vi "1_OnDemand.vi"() -> ()   [LabVIEW 2020]
uses:
  <vilib>/Instr/_visa.llb/VISA Configure Serial Port (Instr).vi
  <vilib>/Analysis/NI_AALBase.lvlib
panel:
  in  "stop":bool
  in  "Tab Control":enum32{"Main", "Service"}(tab)
  out "mean":dbl=672.206 format="%.6f"
  out "standard deviation":dbl=7.149110683653894 format="%.6f"
  out "Measurement":dbl(graph)=673.0
  out "error out":errorcluster
  in  "VISA resource name":refnum<visa-resource-name>="COM7"
  out "answer":string="673 \n\r"
  in  "Clear":bool
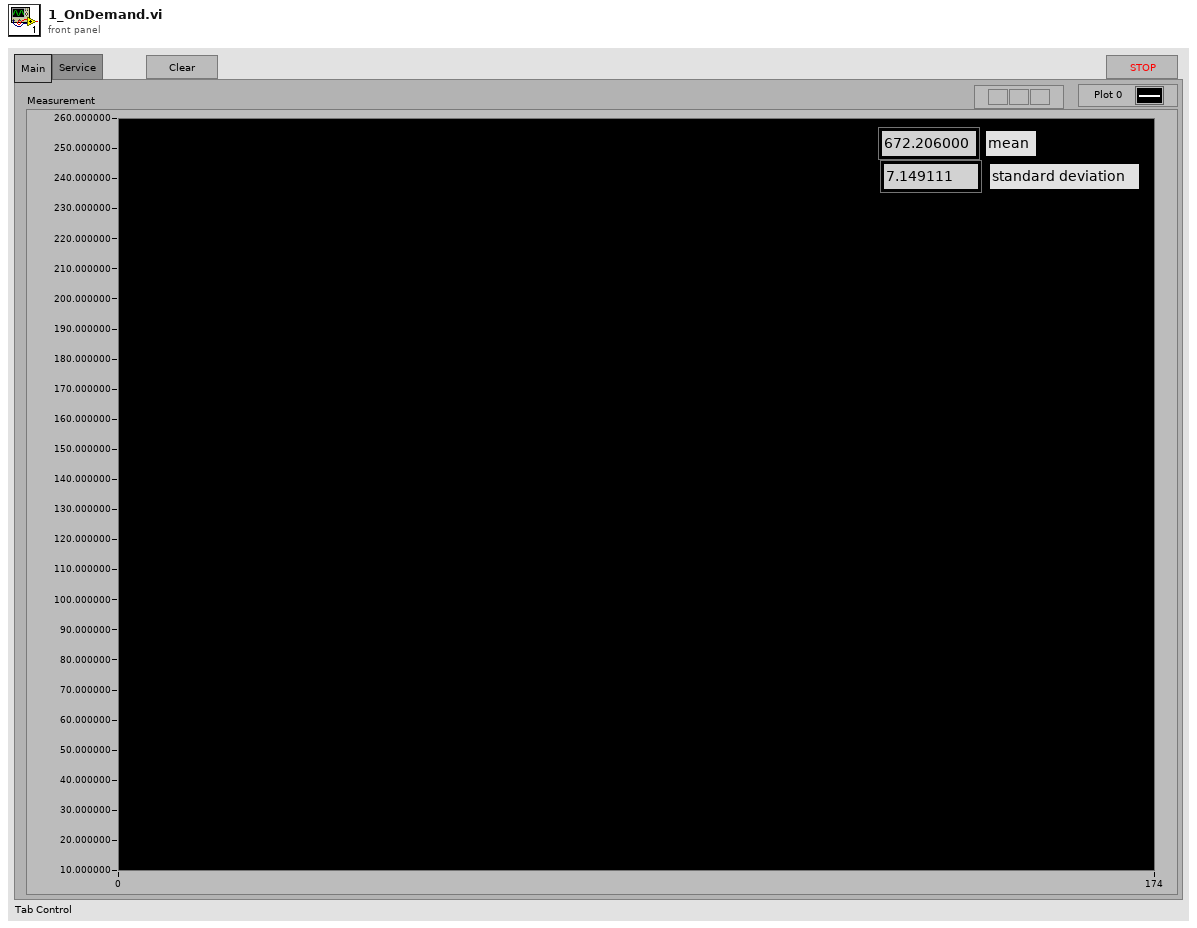
[diagram p1: front panel]
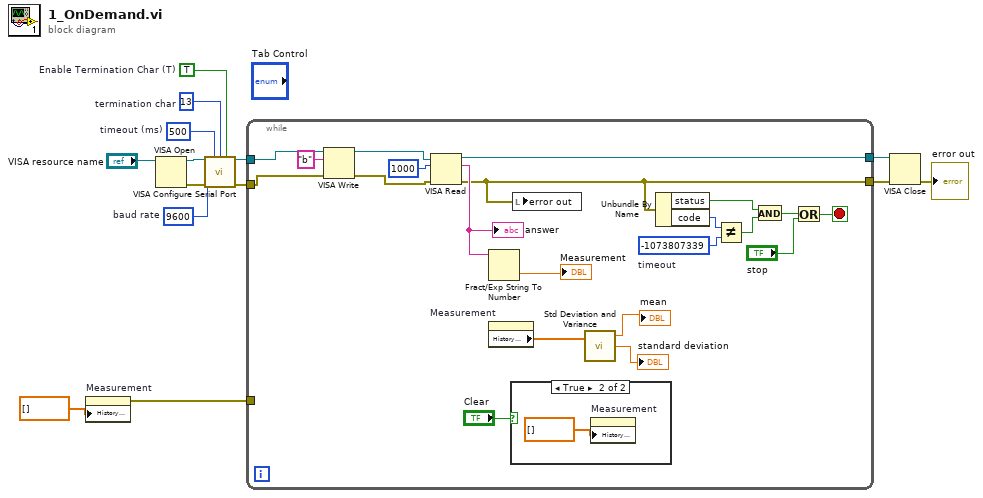
[diagram p0: block diagram]
diagram:
  w3 = u32 9600  # baud rate
  w4 = u32 500  # timeout (ms)
  w10 = TRUE  # Enable Termination Char (T)
  w11 = u8 13  # termination char
  n1 = property on="Measurement" class="WFChart (strict)"("History Data"=dbl[] []) -> (error out=w1:errorcluster)  [unwired: 2 in, 1 out]
  n2 = VISA Open(VISA resource name="VISA resource name") -> (VISA resource name=w13:refnum<visa-resource-name>, error out=w14:errorcluster)  [unwired: 4 in]
  n3 = call-poly "VISA Configure Serial Port"("VISA resource name"=w13, "timeout (10sec)"=w4, "termination char\n(0xA = '\\n' = LF)"=w11, "Enable Termination\nChar (T)"=w10, "baud rate (9600)"=w3, "error in (no error)"=w14) -> ("VISA resource name out"=w7:refnum<visa-resource-name>, "error out"=w6:errorcluster)  [unwired: 8 in]
  n4 = while {
    tunnel: w7 -> [w34]
    tunnel: [w35] -> w9
    tunnel: w6 -> [w16]
    tunnel: [w27] -> w8
    tunnel: w1 -> [_]
    stop <- w21 stop-if-true
    w25 = -1073807339  # timeout
    n5 = VISA Write(VISA resource name=w34, write buffer="b", error in (no error)=w16) -> (VISA resource name out=w18:refnum<visa-resource-name>, error out=w15:errorcluster)  [unwired: 1 out]
    n6 = VISA Read(VISA resource name=w18, byte count=u32 1000, error in (no error)=w15) -> (VISA resource name out=w35:refnum<visa-resource-name>, read buffer=w32:string, error out=w27:errorcluster)  [unwired: 1 out]
    "answer" <- w32
    n7 = Fract/Exp String To Number(string=w32) -> (number=→"Measurement":dbl)  [unwired: 3 in, 1 out]
    n8 = property on="Measurement" class="WFChart (strict)"() -> ("History Data"=w31:dbl[])  [unwired: 2 in, 2 out]
    n9 = case shown="True" "Clear" {
      frame False {
      }
      frame True {
        n10 = property on="Measurement" class="WFChart (strict)"("History Data"=dbl[] []) -> ()  [unwired: 2 in, 2 out]
      }
    }
    n11 = local write "error out"(w27) -> ()
    n12 = call <vilib>:"Std Deviation and Variance.vi"("X"=w31) -> ("mean"=→"mean":dbl, "standard deviation"=→"standard deviation":dbl)  [unwired: 1 in, 1 out]
    n13 = Unbundle By Name(w27) -> ("status"=w23:bool, "code"=w26:i32)
    n14 = Not Equal?(x=w26, y=w25) -> (x != y?=w24:bool)
    n15 = And(x=w23, y=w24) -> (x .and. y?=w22:bool)
    n16 = Or(x=w22, y="stop") -> (x .or. y?=w21:bool)
  }
  n17 = VISA Close(VISA resource name=w9, error in (no error)=w8) -> (error out=→"error out":errorcluster)
